vi "UpdatesToMessages.vi"(0 "reference in":refnum<class "TelegramBOT.lvclass">, 2 "result":T2[](array[typedef]), 5 "error in (no error)":errorcluster) -> (14 "reference out":refnum<class "TelegramBOT.lvclass">, 16 "Messages":T1[](array[typedef]), 19 "error out":errorcluster)   [LabVIEW 2014, in "TelegramBOT.lvclass"]
uses:
  TelegramBOT.lvclass
  UpdateResultElem.ctl
  MessageCluster.ctl
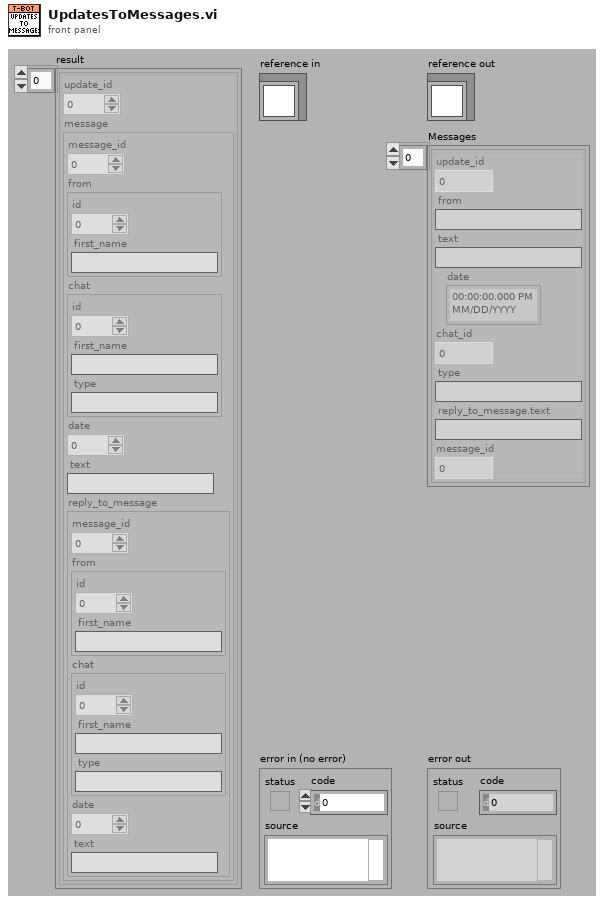
[diagram p1: front panel]
types:
  T1 = typedef "TelegramBOT.lvclass/MessageCluster.ctl" = cluster{"update_id":u32, "from":string, "text":string, "date":timestamp, "chat_id":i32, "type":string, "reply_to_message.text":string, "message_id":u32}
  T2 = typedef "TelegramBOT.lvclass/UpdateResultElem.ctl" = cluster{"update_id":u32, "message":cluster{"message_id":u32, "from":cluster{"id":u64, "first_name":string}, "chat":cluster{"id":i32, "first_name":string, "type":string}, "date":u32, "text":string, "reply_to_message":cluster{"message_id":u32, "from":cluster{"id":u64, "first_name":string}, "chat":cluster{"id":i32, "first_name":string, "type":string}, "date":u32, "text":string}}}
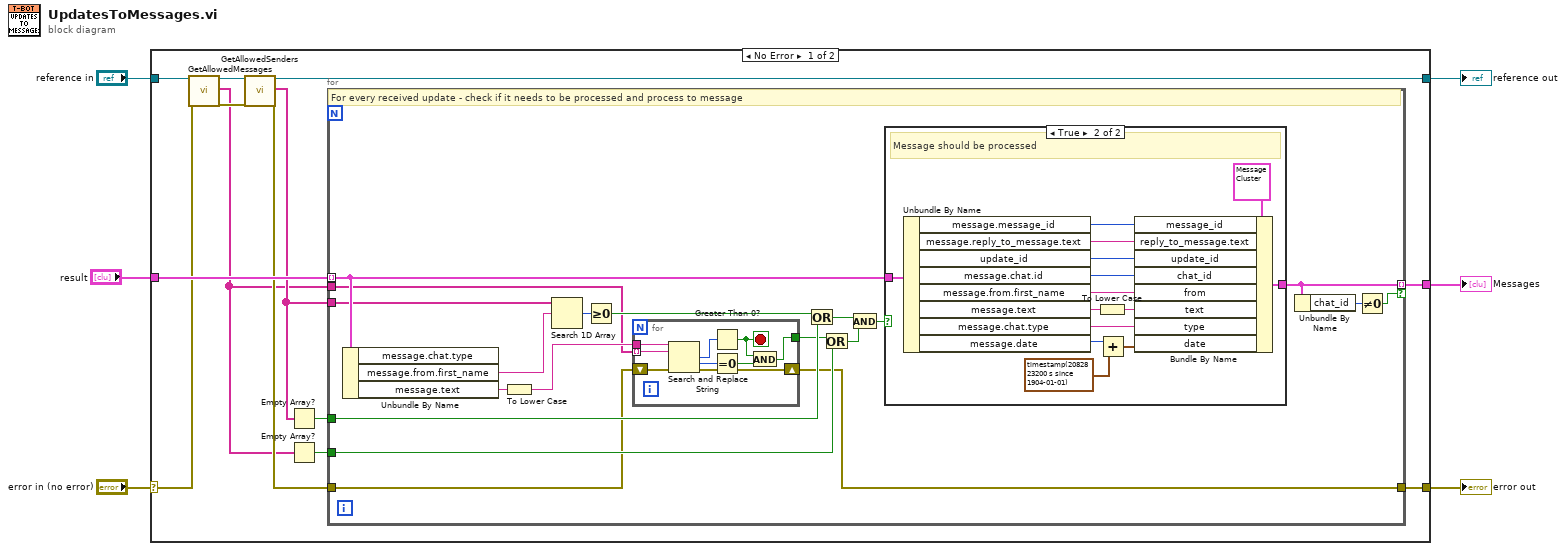
[diagram p0: block diagram]
diagram:
  n1 = case shown="No Error" "error in (no error)" {
    selector: "error in (no error)" -> [w11 w63]
    tunnel: [w19 w63] -> w5
    tunnel: [w13 w62] -> w3
    tunnel: "reference in" -> [w15 w62]
    tunnel: "result" -> [w18 _]
    tunnel: [w17 _] -> w1
    frame No Error {
      n2 = call "GetAllowedMessages.vi"("reference in"=w15, "error in (no error)"=w11) -> ("reference out"=w14:refnum<class "TelegramBOT.lvclass">, "AllowedMessages"=w7:string[], "error out"=w12:errorcluster)  [unwired: 15 in]
      n3 = call "GetAllowedSenders.vi"("reference in"=w14, "error in (no error)"=w12) -> ("reference out"=w13:refnum<class "TelegramBOT.lvclass">, "AllowedSenders"=w8:string[], "error out"=w9:errorcluster)  [unwired: 15 in]
      n4 = Empty Array?(array=w8) -> (empty?=w16:bool)
      n5 = Empty Array?(array=w7) -> (empty?=w10:bool)
      n6 = for {
        tunnel: w18 -> [w33] mode=indexing
        tunnel: w16 -> [w35]
        tunnel: w10 -> [w26]
        tunnel: [w29] -> w17 mode=indexing if=w27
        tunnel: w9 -> [w24]
        tunnel: [w25] -> w19
        tunnel: w8 -> [w21]
        tunnel: w7 -> [w20]
        # "For every received update - check if it needs to be processed and process to message"
        n7 = Unbundle By Name(w33) -> ("message.from.first_name"=w37:string, "message.text"=w23:string)  [unwired: 1 out]
        n8 = To Lower Case(string=w23) -> (all lower case string=w22:string)
        n9 = Search 1D Array(1D array=w21, element=w37) -> (index of element=w38:i32)  [unwired: 1 in]
        n10 = Greater Or Equal To 0?(x=w38) -> (x >= 0?=w36:bool)
        n11 = for {
          tunnel: w20 -> [w61] mode=indexing
          tunnel: [w56] -> w32
          tunnel: w22 -> [w59]
          shift-right: [w54] -> w25
          shift-left: w24 -> [w53]
          stop <- w55 stop-if-true
          n12 = Search and Replace String(input string=w59, search string=w61, error in=w53) -> (number of replacements=w60:i32, offset past replacement=w58:i32, error out=w54:errorcluster)  [unwired: 5 in, 1 out]
          n13 = Greater Than 0?(x=w60) -> (x > 0?=w55:bool)
          n14 = Equal To 0?(x=w58) -> (x = 0?=w57:bool)
          n15 = And(x=w55, y=w57) -> (x .and. y?=w56:bool)
        }
        n16 = Or(x=w36, y=w35) -> (x .or. y?=w31:bool)
        n17 = Or(x=w32, y=w26) -> (x .or. y?=w30:bool)
        n18 = And(x=w31, y=w30) -> (x .and. y?=w34:bool)
        n19 = case shown="True" w34 {
          tunnel: w33 -> [_ w45]
          tunnel: [_ w41] -> w29
          frame False {
            # "Message ignored"
          }
          frame True {
            # "Message should be processed"
            n20 = Unbundle By Name(w45) -> ("message.message_id"=w42:u32, "message.reply_to_message.text"=w44:string, "update_id"=w46:u32, "message.chat.id"=w50:i32, "message.from.first_name"=w47:string, "message.text"=w40:string, "message.chat.type"=w52:string, "message.date"=w48:u32)
            n21 = To Lower Case(string=w40) -> (all lower case string=w39:string)
            n22 = Add(x=w48, y=timestamp(2082823200 s since 1904-01-01)) -> (x+y=w49:timestamp)
            n23 = Bundle By Name(cluster=T1 {"update_id"=0, "from"="", "text"="", "date"=timestamp(0 s since 1904-01-01), "chat_id"=0, "type"="", "reply_to_message.text"="", "message_id"=0} ("Message"), "message_id"=w42, "reply_to_message.text"=w44, "update_id"=w46, "chat_id"=w50, "from"=w47, "text"=w39, "type"=w52, "date"=w49) -> (w41:T1)
          }
        }
        n24 = Unbundle By Name(w29) -> ("chat_id"=w28:i32)
        n25 = Not Equal To 0?(x=w28) -> (x != 0?=w27:bool)
      }
    }
    frame Error {
    }
  }
  "error out" <- w5
  "reference out" <- w3
  "Messages" <- w1
